vi "Bezahl_simulation.vi"(8 "error in":errorcluster) -> (0 "error out":errorcluster, 2 "Betrag erreicht":bool)   [LabVIEW 2023]
uses:
  CONTROLS/FGV-status.ctl
panel:
  out "Restgeldbetrag":dbl
  in  "Storno":bool
  out "Guthaben":dbl
  out "Preis":dbl
  in  "100 Euro":bool
  in  "50 Euro":bool
  in  "20 Euro":bool
  in  "10 Euro":bool
  in  "1 Euro":bool
  in  "2 Euro":bool
  in  "Bezahlen":bool
  in  "5 Euro":bool
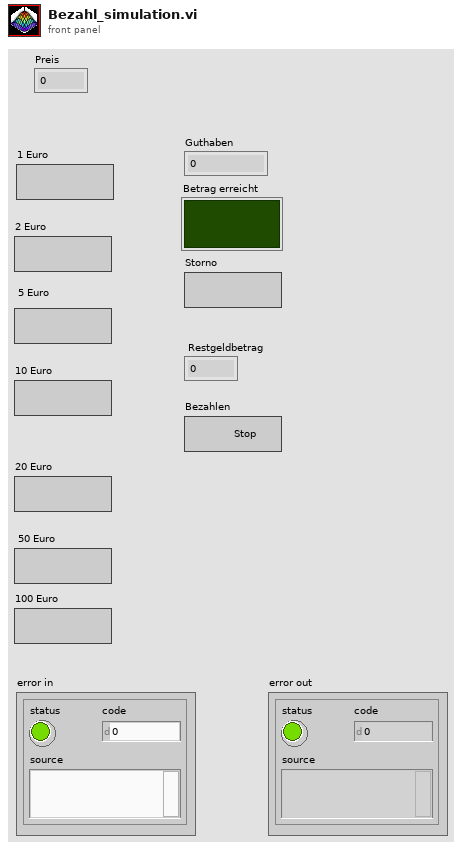
[diagram p1: front panel]
types:
  T1 = typedef "FGV-status.ctl" = enum16{"Read", "Write"}
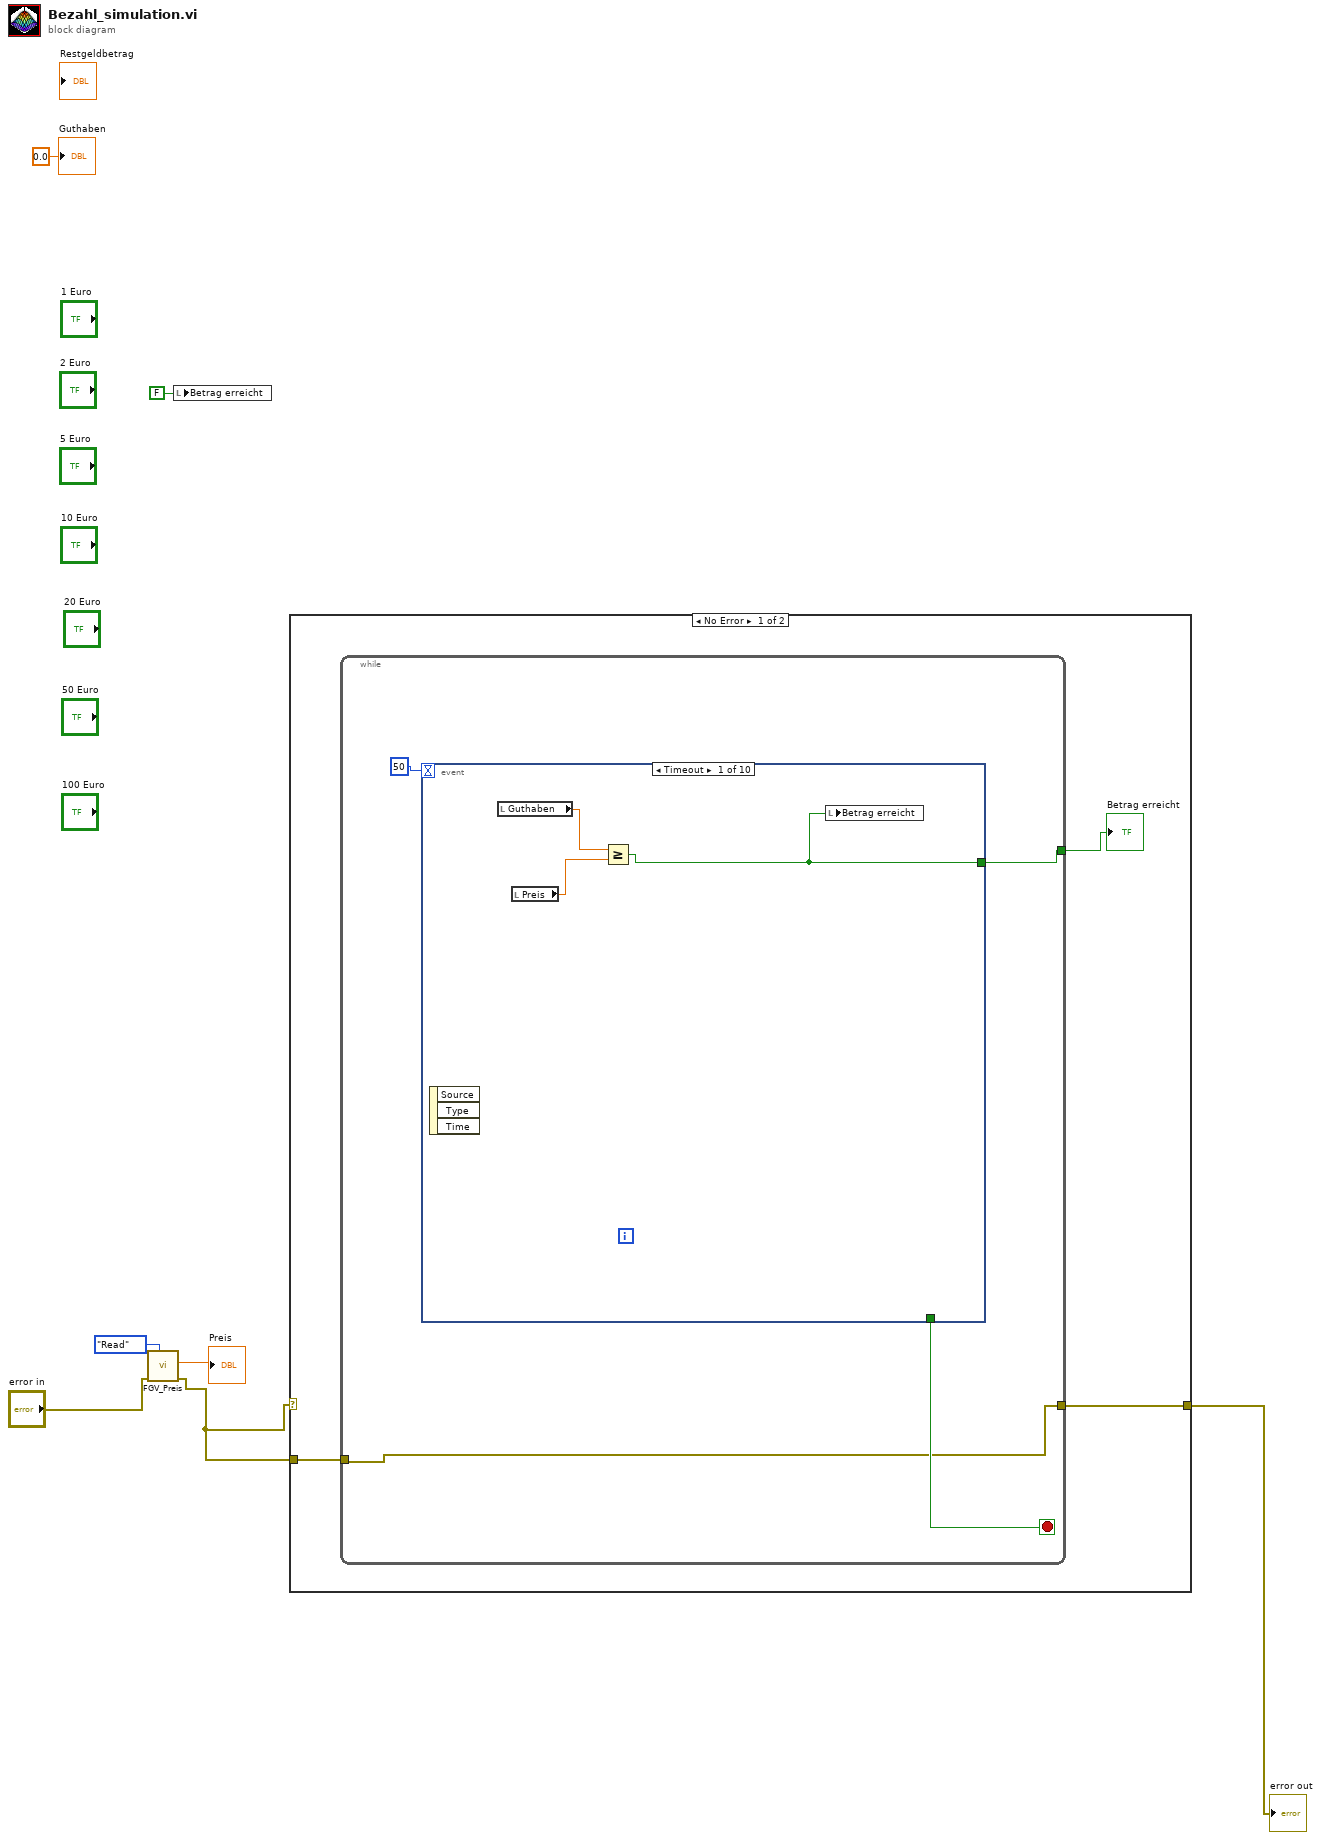
[diagram p0: block diagram]
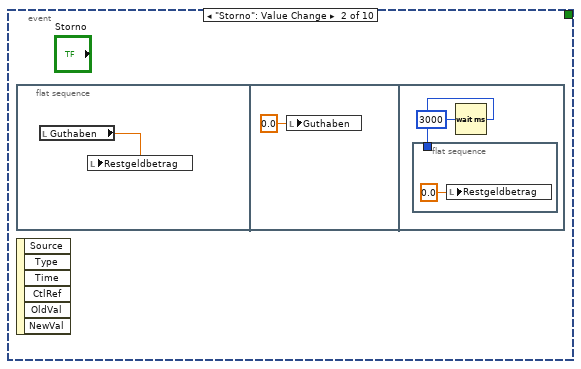
[diagram p2: hidden frame]
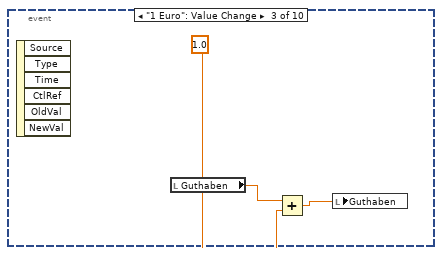
[diagram p3: hidden frame]
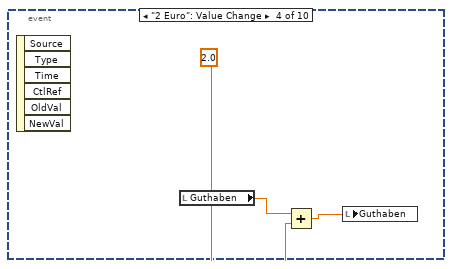
[diagram p4: hidden frame]
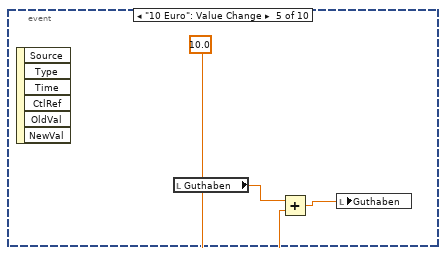
[diagram p5: hidden frame]
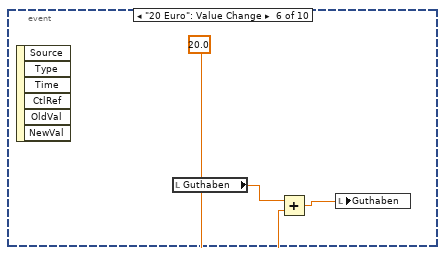
[diagram p6: hidden frame]
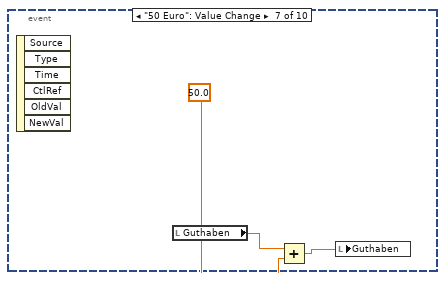
[diagram p7: hidden frame]
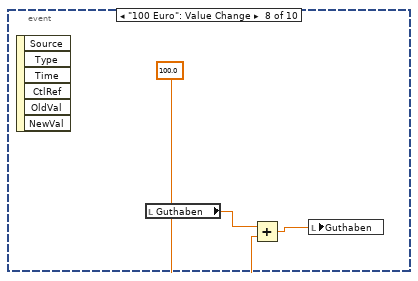
[diagram p8: hidden frame]
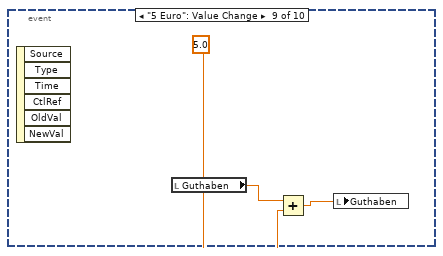
[diagram p9: hidden frame]
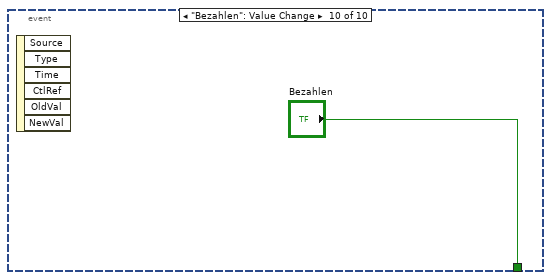
[diagram p10: hidden frame]
diagram:
  n1 = call "FGV_Preis.vi"("fgv-Status"=FGV-status."Read", "error in (no error)"="error in") -> ("error out"=w2:errorcluster, "Preis Output"=→"Preis":dbl)  [unwired: 8 in]
  n2 = local write "Betrag erreicht"(FALSE ("Betrag erreicht")) -> ()
  n3 = case shown="No Error" w2 {
    tunnel: w2 -> [w10 w45]
    tunnel: [w8 w45] -> w5
    frame No Error {
      n4 = while {
        tunnel: [w13] -> w9
        tunnel: w10 -> [w11]
        tunnel: [w11] -> w8
        stop <- w14 stop-if-true
        n5 = event shown="[0] Timeout" {
          selector: _ -> [_ _ _ _ _ _ _ _ _ _]
          dyn-events: _ -> [_ _ _ _ _ _ _ _ _ _]
          timeout: 50 -> [_ _ _ _ _ _ _ _ _ _]
          tunnel: [_ _ _ _ _ _ _ _ _ "Bezahlen"] -> w14
          tunnel: [w15 _ _ _ _ _ _ _ _ _] -> w13
          event Timeout {
            n6 = event-data() -> ()  [unwired: 1 in, 3 out]
            n7 = local read "Guthaben"() -> (w17:dbl)
            n8 = local read "Preis"() -> (w16:dbl)
            n9 = Greater Or Equal?(x=w17, y=w16) -> (x >= y?=w15:bool)
            n10 = local write "Betrag erreicht"(w15) -> ()
          }
          event "Storno": Value Change {
            n11 = flat-sequence {
              frame #0 {
                n12 = local read "Guthaben"() -> (w18:dbl)
                n13 = local write "Restgeldbetrag"(w18) -> ()
              }
              frame #1 {
                n14 = local write "Guthaben"(0.0 ("Guthaben")) -> ()
              }
              frame #2 {
                n15 = flat-sequence {
                  tunnel: w21 -> [_]
                  frame #0 {
                    n16 = local write "Restgeldbetrag"(0.0 ("Restgeldbetrag")) -> ()
                  }
                }
                n17 = Wait (ms)(milliseconds to wait=u32 3000) -> (millisecond timer value=w21:u32)
              }
            }
            n18 = event-data() -> ()  [unwired: 1 in, 6 out]
          }
          event "1 Euro": Value Change {
            n19 = event-data() -> ()  [unwired: 1 in, 6 out]
            n20 = local read "Guthaben"() -> (w23:dbl)
            n21 = Add(x=w23, y=1.0 ("Guthaben")) -> (x+y=w25:dbl)
            n22 = local write "Guthaben"(w25) -> ()
          }
          event "2 Euro": Value Change {
            n23 = event-data() -> ()  [unwired: 1 in, 6 out]
            n24 = local read "Guthaben"() -> (w26:dbl)
            n25 = Add(x=w26, y=2.0 ("Guthaben")) -> (x+y=w28:dbl)
            n26 = local write "Guthaben"(w28) -> ()
          }
          event "10 Euro": Value Change {
            n27 = event-data() -> ()  [unwired: 1 in, 6 out]
            n28 = local read "Guthaben"() -> (w29:dbl)
            n29 = Add(x=w29, y=10.0 ("Guthaben")) -> (x+y=w31:dbl)
            n30 = local write "Guthaben"(w31) -> ()
          }
          event "20 Euro": Value Change {
            n31 = event-data() -> ()  [unwired: 1 in, 6 out]
            n32 = local read "Guthaben"() -> (w32:dbl)
            n33 = Add(x=w32, y=20.0 ("Guthaben")) -> (x+y=w34:dbl)
            n34 = local write "Guthaben"(w34) -> ()
          }
          event "50 Euro": Value Change {
            n35 = event-data() -> ()  [unwired: 1 in, 6 out]
            n36 = local read "Guthaben"() -> (w35:dbl)
            n37 = Add(x=w35, y=50.0 ("Guthaben")) -> (x+y=w37:dbl)
            n38 = local write "Guthaben"(w37) -> ()
          }
          event "100 Euro": Value Change {
            n39 = event-data() -> ()  [unwired: 1 in, 6 out]
            n40 = local read "Guthaben"() -> (w38:dbl)
            n41 = Add(x=w38, y=100.0 ("Guthaben")) -> (x+y=w40:dbl)
            n42 = local write "Guthaben"(w40) -> ()
          }
          event "5 Euro": Value Change {
            n43 = event-data() -> ()  [unwired: 1 in, 6 out]
            n44 = local read "Guthaben"() -> (w41:dbl)
            n45 = Add(x=w41, y=5.0 ("Guthaben")) -> (x+y=w43:dbl)
            n46 = local write "Guthaben"(w43) -> ()
          }
          event "Bezahlen": Value Change {
            n47 = event-data() -> ()  [unwired: 1 in, 6 out]
          }
        }
      }
      "Betrag erreicht" <- w9
    }
    frame Error {
    }
  }
  "error out" <- w5
  "Guthaben" <- 0.0 ("Guthaben")
